vi "InitStreamTypeDef.vi"(9 "DAQ Node Array":string[](array[string]), 10 "DAQ Node Count":i32, 11 "StreamTypeDef":T3) -> (3 "StreamTypeDef":T2(array[cluster]))   [LabVIEW 2024]
uses:
  Control/StreamTypeDef.ctl
  Control/streamIO_states.ctl
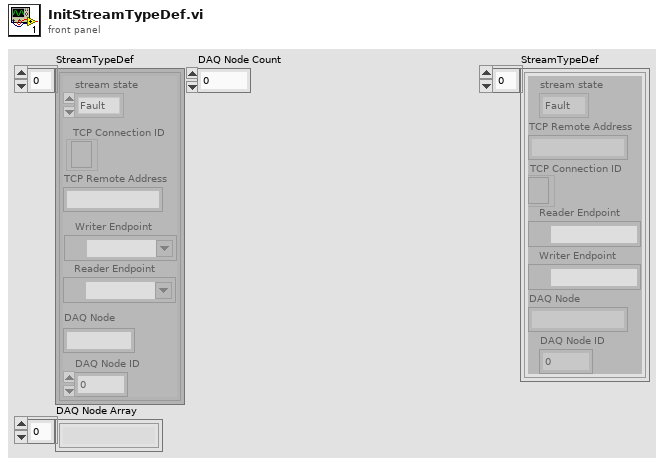
[diagram p1: front panel]
types:
  T1 = typedef "streamIO_states.ctl" = enum16{"Fault", "Initilize", "Stream", "Close"}
  T2 = cluster{"stream state":T1, "TCP Remote Address":string, "TCP Connection ID":refnum<k5>, "Reader Endpoint":refnum<k21>, "Writer Endpoint":refnum<k21>, "DAQ Node":string, "DAQ Node ID":i32}[]
  T3 = typedef "StreamTypeDef.ctl" = cluster{"stream state":T1, "TCP Remote Address":string, "TCP Connection ID":refnum<k5>, "Reader Endpoint":refnum<k21>, "Writer Endpoint":refnum<k21>, "DAQ Node":string, "DAQ Node ID":i32}[]
  T4 = cluster{"stream state":T1, "TCP Remote Address":string, "TCP Connection ID":refnum<k5>, "Reader Endpoint":refnum<k21>, "Writer Endpoint":refnum<k21>, "DAQ Node":string, "DAQ Node ID":i32}
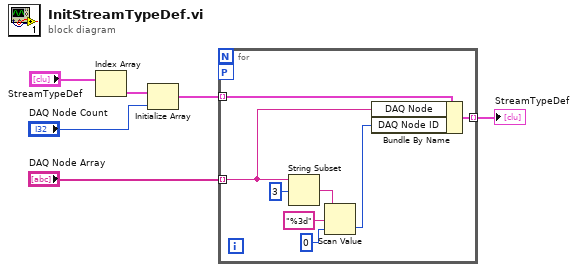
[diagram p0: block diagram]
diagram:
  n1 = Index Array(array="StreamTypeDef") -> (element=w6:T4)  [unwired: 1 in]
  n2 = Initialize Array(w6, "DAQ Node Count") -> (w2:T2)
  n3 = for {
    workers-P: _ -> [_]
    tunnel: "DAQ Node Array" -> [w9] mode=indexing
    tunnel: w2 -> [w10] mode=indexing
    tunnel: [w7] -> w1 mode=indexing
    n4 = String Subset(string=w9, offset (0)=3) -> (substring=w14:string)  [unwired: 1 in]
    n5 = Scan Value(string=w14, format string="%3d", default (0 dbl)=0) -> (value=w8:i32)  [unwired: 1 out]
    n6 = Bundle By Name(cluster=w10, "DAQ Node"=w9, "DAQ Node ID"=w8) -> (w7:T4)
  }
  "StreamTypeDef" <- w1
